vi "Arbitary.vi"() -> ()   [LabVIEW 2013]
uses:
  <vilib>/Analysis/NI_AALBase.lvlib
panel:
  in  "stop":bool
  in  "Frequency Unit":u16(ring) items=["Hz", "cycles"]
  in  "Reset phase":bool
  in  "Sampling rate (Hz)":dbl(knob)=100.0 step=1.0 scale=0.0..10.0
  in  "Frequency":dbl(knob)=2.01 step=1.0 scale=0.0..10.0
  out "Waveform Pattern":dbl[](graph)
  out "Signal Generated":T1(graph)={0.0, 0.01, "arbitrary wave"=[]}
  in  "interpolation":i32(ring)=1 items=["none", "linear"]
  in  "Wave Table":dbl[](array[knob])=[0.0, 1.0, 4.0, 0.2, -0.9] scale=0.0..10.0
  in  "Amplitude":dbl(knob)=3.7755102040816326 scale=0.0..5.0
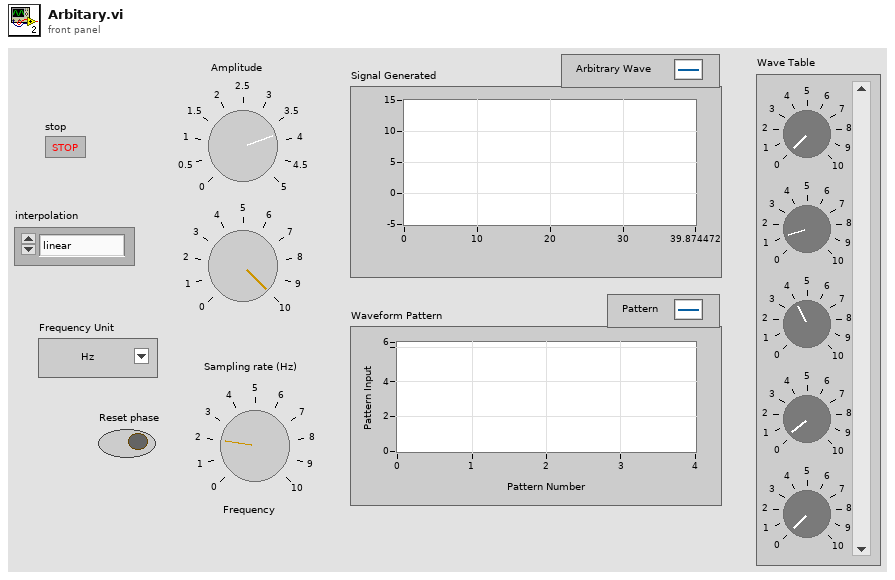
[diagram p1: front panel]
types:
  T1 = cluster{dbl[unit], dbl[unit], "arbitrary wave":dbl[]}
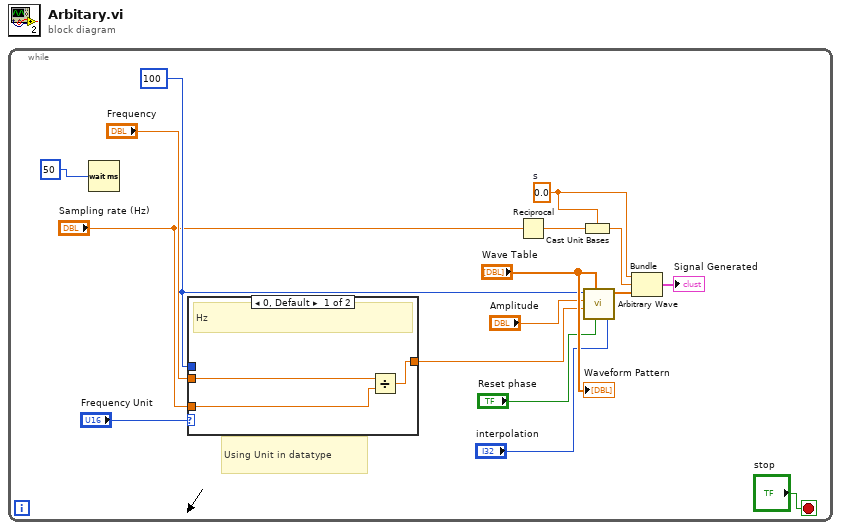
[diagram p0: block diagram]
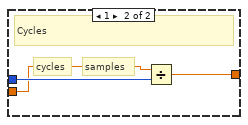
[diagram p2: hidden frame]
diagram:
  n1 = while {
    stop <- "stop" stop-if-true
    w4 = dbl[unit] 0.0  # s
    w14 = 100 ("samples")
    # "Using Unit in datatype"
    n2 = Wait (ms)(milliseconds to wait=u32 50) -> ()  [unwired: 1 out]
    n3 = case shown="0, Default" "Frequency Unit" {
      tunnel: [w19 w21] -> w2
      tunnel: w14 -> [_ w22]
      tunnel: "Frequency" -> [w18 w20]
      tunnel: "Sampling rate (Hz)" -> [w17 _]
      frame 0, Default {
        # "Hz"
        n4 = Divide(x=w18, y=w17) -> (x/y=w19:dbl)
      }
      frame 1 {
        # "samples"
        # "cycles"
        # "Cycles"
        n5 = Divide(x=w20, y=w22) -> (x/y=w21:dbl)
      }
    }
    n6 = Reciprocal(x="Sampling rate (Hz)") -> (1/x=w8:dbl)
    n7 = Cast Unit Bases(0:w8, 1:w4) -> (2:w7:dbl[unit])
    n8 = call <vilib>:"Arbitrary Wave.vi"("interpolation"="interpolation", "reset phase"="Reset phase", "Wave Table"="Wave Table", "frequency"=w2, "amplitude"="Amplitude", "samples"=w14) -> ("arbitrary wave"=w10:dbl[])  [unwired: 1 in, 2 out]
    n9 = Bundle(w4, w7, "arbitrary wave"=w10) -> (→"Signal Generated":T1)  [unwired: 1 in]
    "Waveform Pattern" <- "Wave Table"
  }
